vi "Saveissue.vi"() -> ()   [LabVIEW 2011]
panel:
  out "Acquiring Data":bool
  in  "Cancel Acquisition":bool caption="Cancel\nAcquisition"
  in  "Horizontal bin":i32=1
  in  "Vertical bin":i32=1
  in  "Number in series":i32=3
  out "Calculated Exposure Value":sgl format="%.4f"
  out "Return from CheckTimings":u32
  in  "Stop":bool
  in  "Time between captures (s)":dbl
  in  "Number of captures":i32=1
  in  "Run Kinetic":bool caption="Run\nKinetic"
  in  "Start Delay (s)":u32
  out "Image Array":i32[](array[numeric]) caption="Array"
  out "Intensity Graph":i32[][](graph)
  out "SetTriggerMode":u32
  out "SetVSSpeed":u32
  out "SetHSSpeed":u32
  out "SetExposureTime":u32
  in  "Exposure Time (secs)":sgl=0.1 format="%.2f"
  out "SetImage":u32
  out "SetReadMode":u32
  out "SetAcquisition Mode":u32
  out "X Pixels":i32
  out "Y Pixels":i32
  out "GetDetector":u32
  out "Total number of pixels":i32
  out "error out":errorcluster
  in  "Base Path":path=path "D:/Andor/data"
  in  "File Name":string="test"
  in  "File #":i32=1
  out "Sample Output File":string="D:\\Andor\\data\\test_1.sif"
  out "Current":i32 caption="Current Capture Number"
  out "Next Image Time":timestamp
  in  "error in (no error)":errorcluster
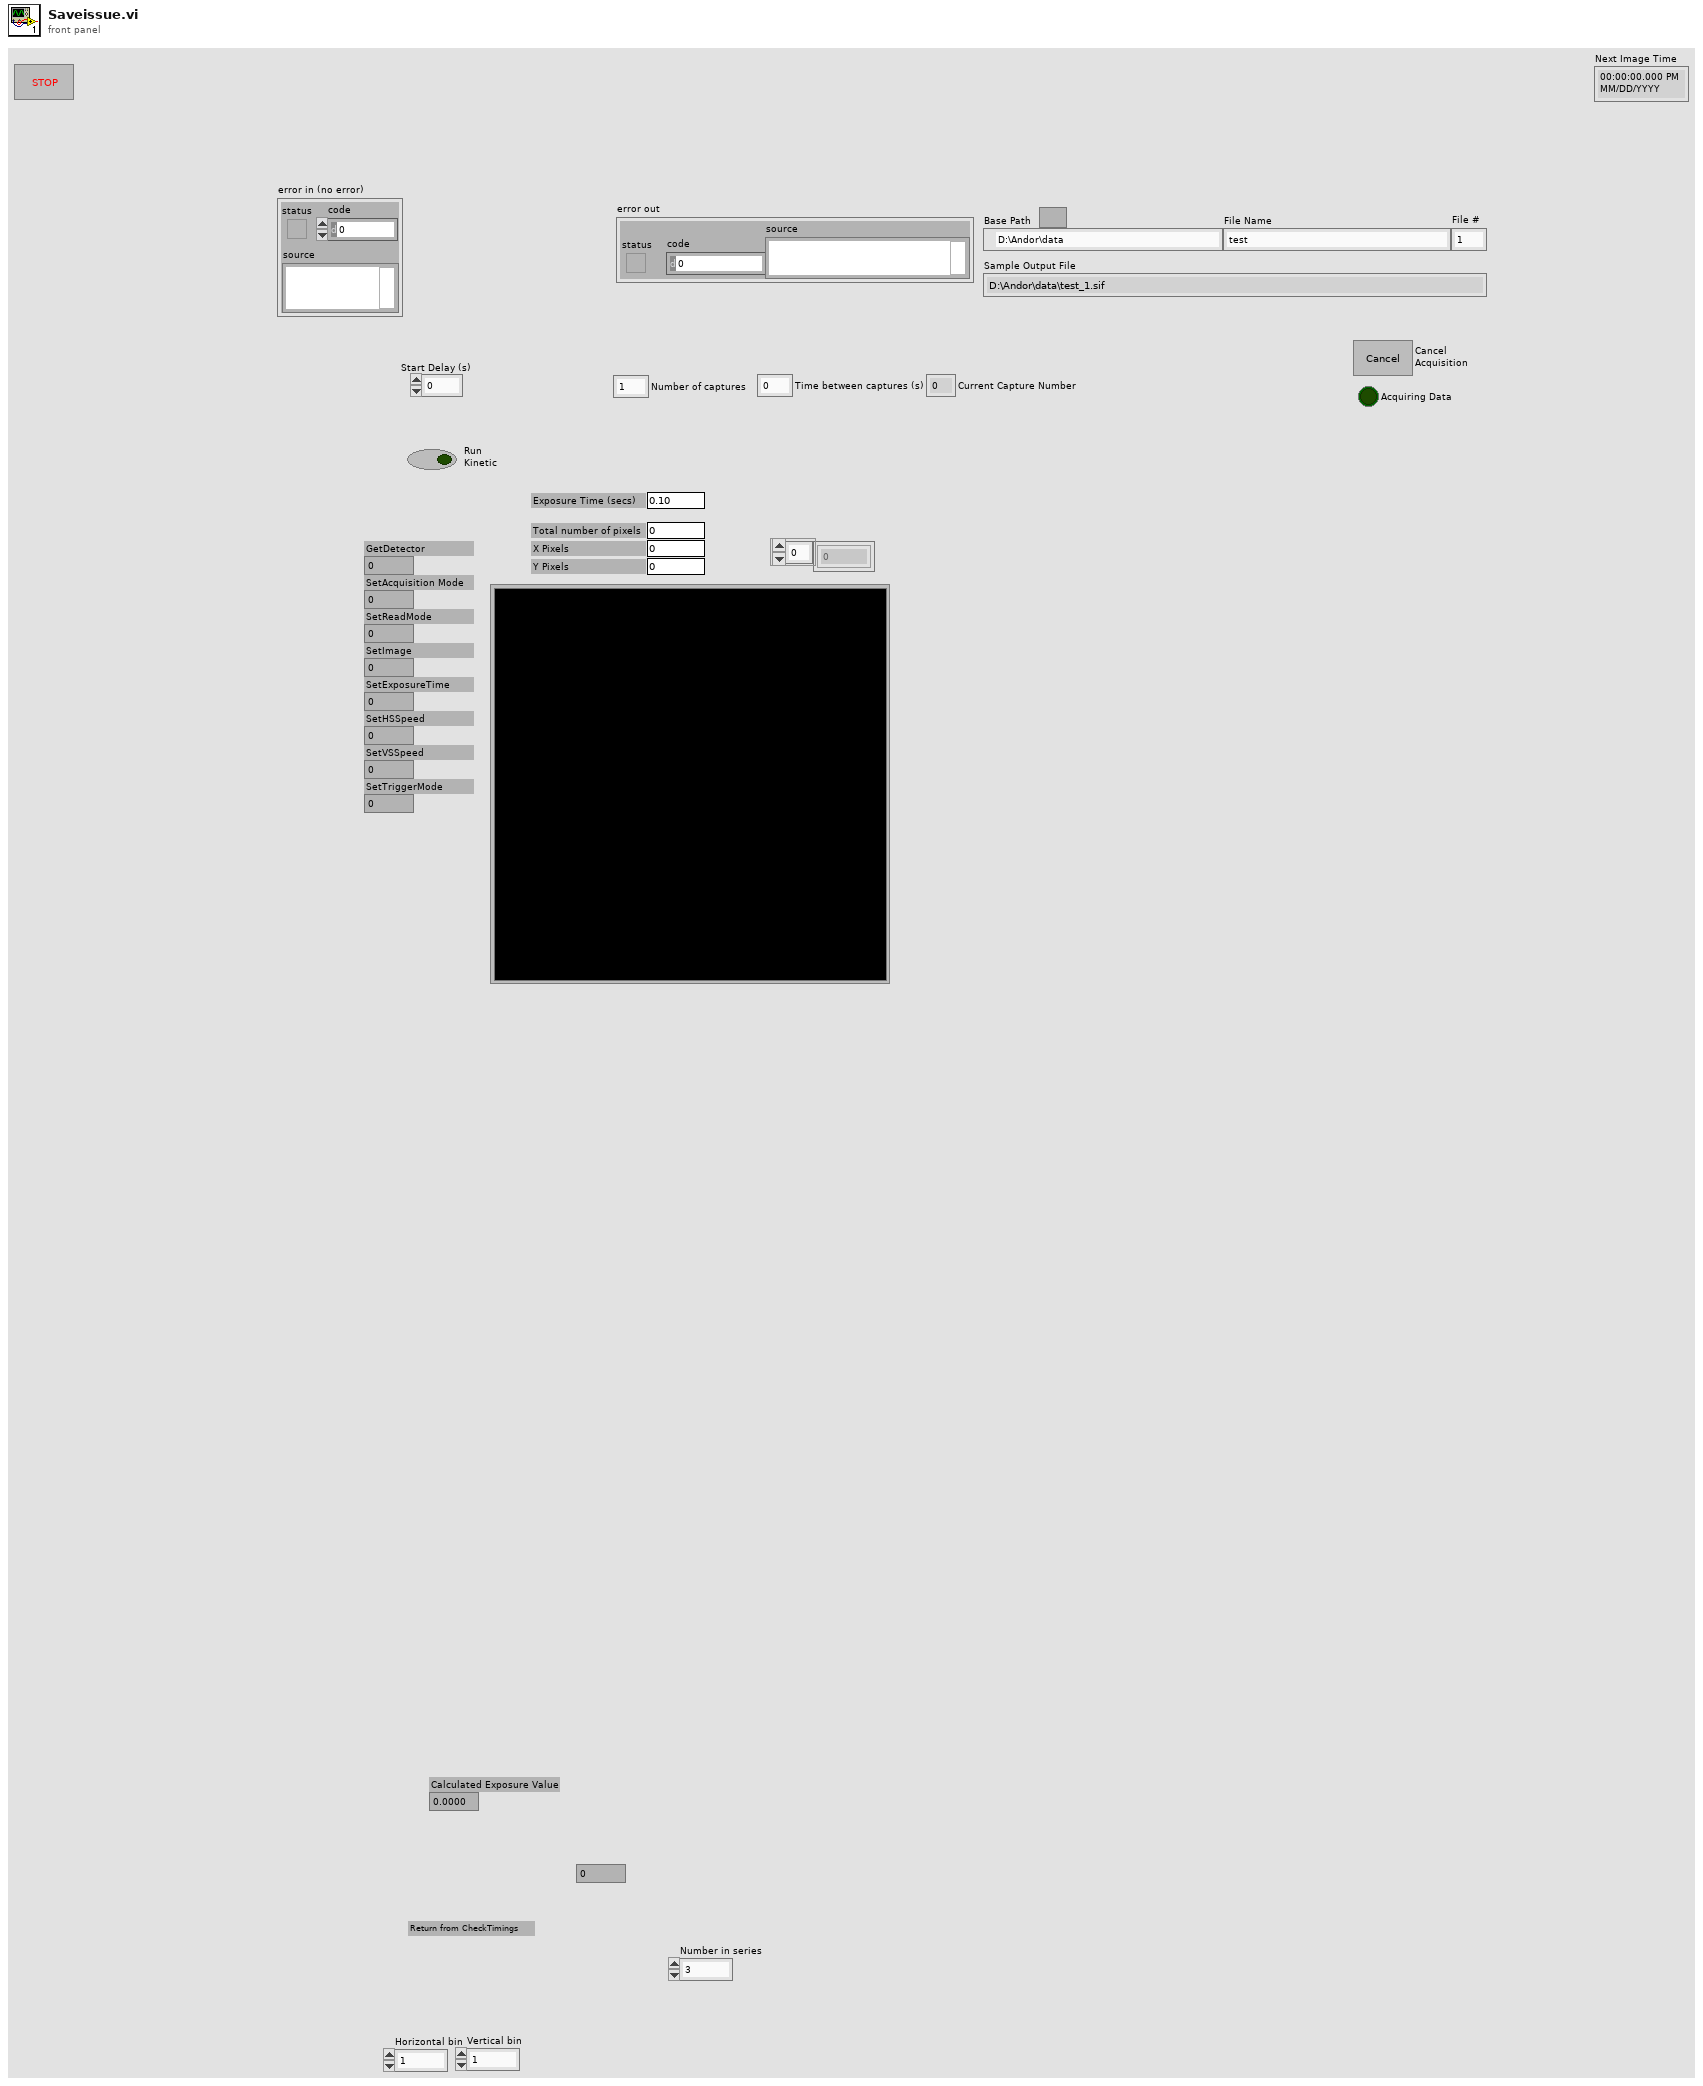
[diagram p1: front panel]
types:
  T1 = typedef "Error Code Enum typedef.ctl" = enum32{"N/A (0)", "DRV_ERROR_CODES", "DRV_SUCCESS", "DRV_VXDNOTINSTALLED", "DRV_ERROR_SCAN", "DRV_ERROR_CHECK_SUM", "DRV_ERROR_FILELOAD", "DRV_UNKNOWN_FUNC", "DRV_ERROR_VXD_INIT", "DRV_ERROR_ADDRESS", "DRV_ERROR_PAGELOCK", "DRV_ERROR_PAGEUNLOCK", "DRV_ERROR_BOARDTEST", "DRV_ERROR_ACK", "DRV_ERROR_UP_FIFO", "DRV_ERROR_PATTERN", "N/A (16)", "DRV_ACQUISITION_ERRORS", "DRV_ACQ_BUFFER", "DRV_ACQ_DOWNFIFO_FULL", "DRV_PROC_UNKONWN_INSTRUCTION", "DRV_ILLEGAL_OP_CODE", "DRV_KINETIC_TIME_NOT_MET", "DRV_ACCUM_TIME_NOT_MET", "DRV_NO_NEW_DATA", "N/A (25)", "DRV_SPOOLERROR", "N/A (27)", "N/A (28)", "N/A (29)", "N/A (30)", "N/A (31)", "N/A (32)", "DRV_TEMPERATURE_CODES", "DRV_TEMPERATURE_OFF", "DRV_TEMPERATURE_NOT_STABILIZED", "DRV_TEMPERATURE_STABILIZED", "DRV_TEMPERATURE_NOT_REACHED", "DRV_TEMPERATURE_OUT_RANGE", "DRV_TEMPERATURE_NOT_SUPPORTED", "DRV_TEMPERATURE_DRIFT", "N/A (41)", "N/A (42)", "N/A (43)", "N/A (44)", "N/A (45)", "N/A (46)", "N/A (47)", "N/A (48)", "DRV_GENERAL_ERRORS", "DRV_INVALID_AUX", "DRV_COF_NOTLOADED", "DRV_FPGAPROG", "DRV_FLEXERROR", "DRV_GPIBERROR", "N/A (55)", "N/A (56)", "N/A (57)", "N/A (58)", "N/A (59)", "N/A (60)", "N/A (61)", "N/A (62)", "N/A (63)", "DRV_DATATYPE", "DRV_DRIVER_ERRORS", "DRV_P1INVALID", "DRV_P2INVALID", "DRV_P3INVALID", "DRV_P4INVALID", "DRV_INIERROR", "DRV_COFERROR", "DRV_ACQUIRING", "DRV_IDLE", "DRV_TEMPCYCLE", "DRV_NOT_INITIALIZED", "DRV_P5INVALID", "DRV_P6INVALID", "DRV_INVALID_MODE", "DRV_INVALID_FILTER", "DRV_I2CERRORS", "DRV_I2CDEVNOTFOUND", "DRV_I2CTIMEOUT", "DRV_P7INVALID", "N/A (84)", "N/A (85)", "N/A (86)", "N/A (87)", "N/A (88)", "N/A (89)", "DRV_IOCERROR", "DRV_VRMVERSIONERROR"}
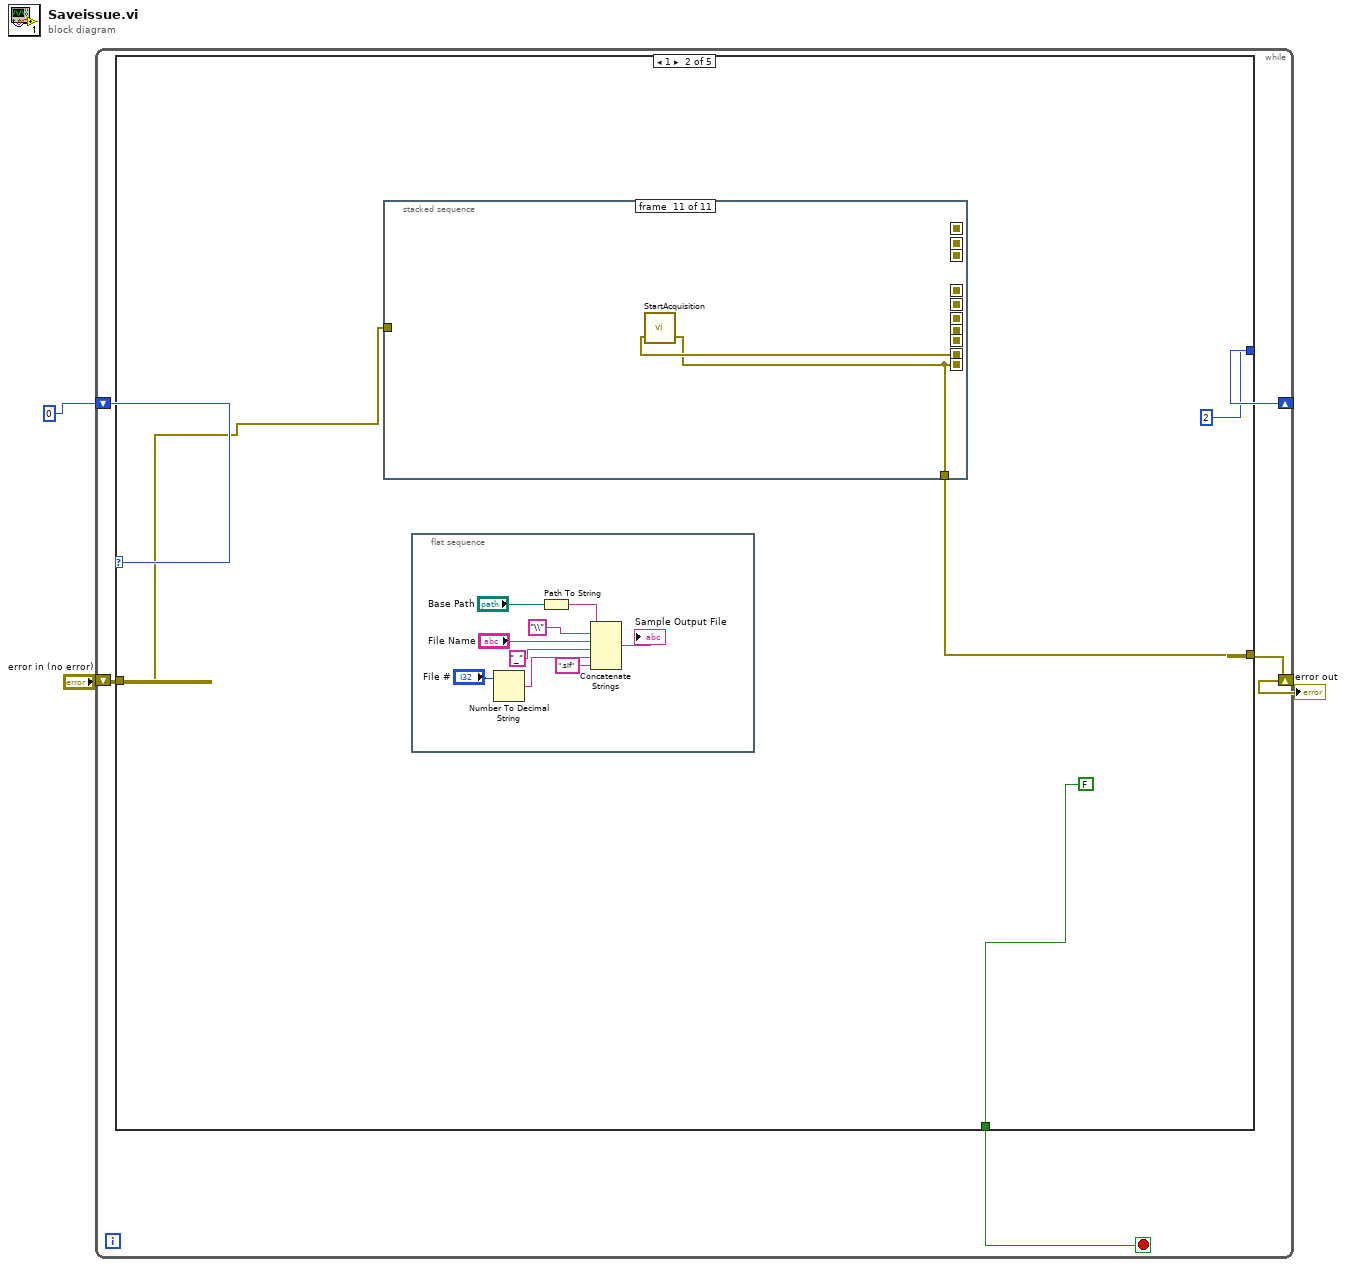
[diagram p0: block diagram]
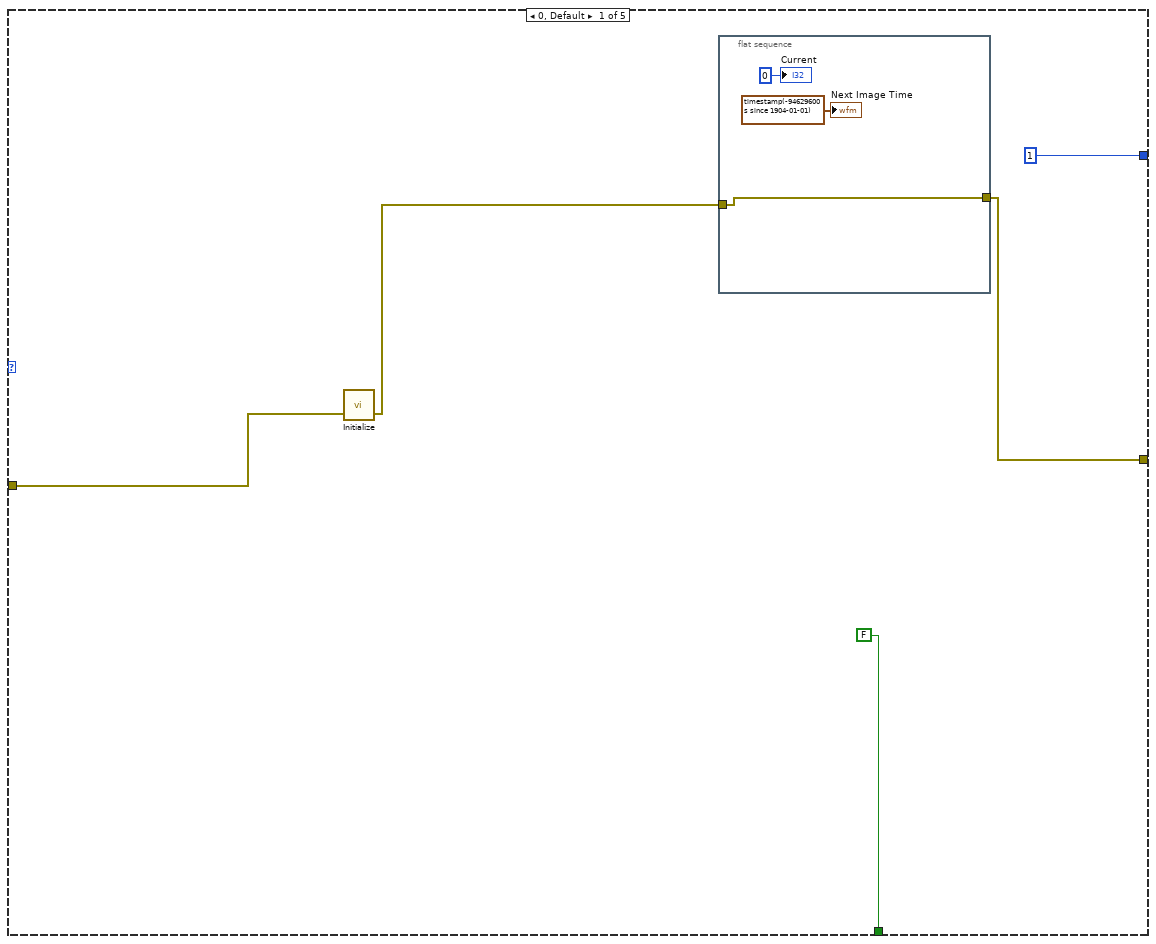
[diagram p2: hidden frame]
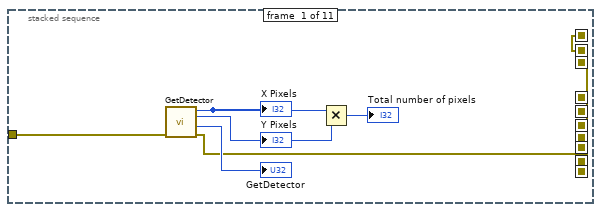
[diagram p3: hidden frame]
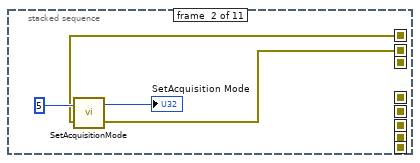
[diagram p4: hidden frame]
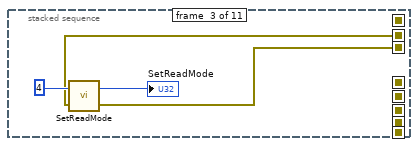
[diagram p5: hidden frame]
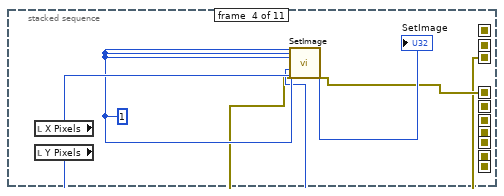
[diagram p6: hidden frame]
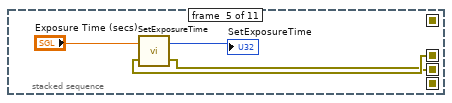
[diagram p7: hidden frame]
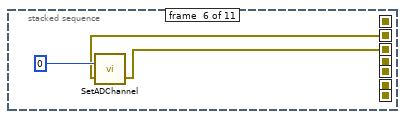
[diagram p8: hidden frame]
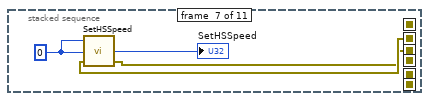
[diagram p9: hidden frame]
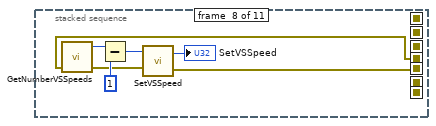
[diagram p10: hidden frame]
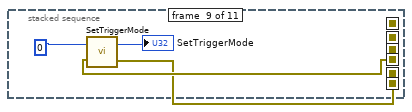
[diagram p11: hidden frame]
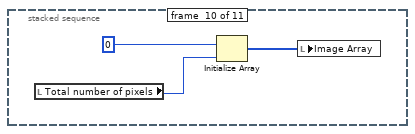
[diagram p12: hidden frame]
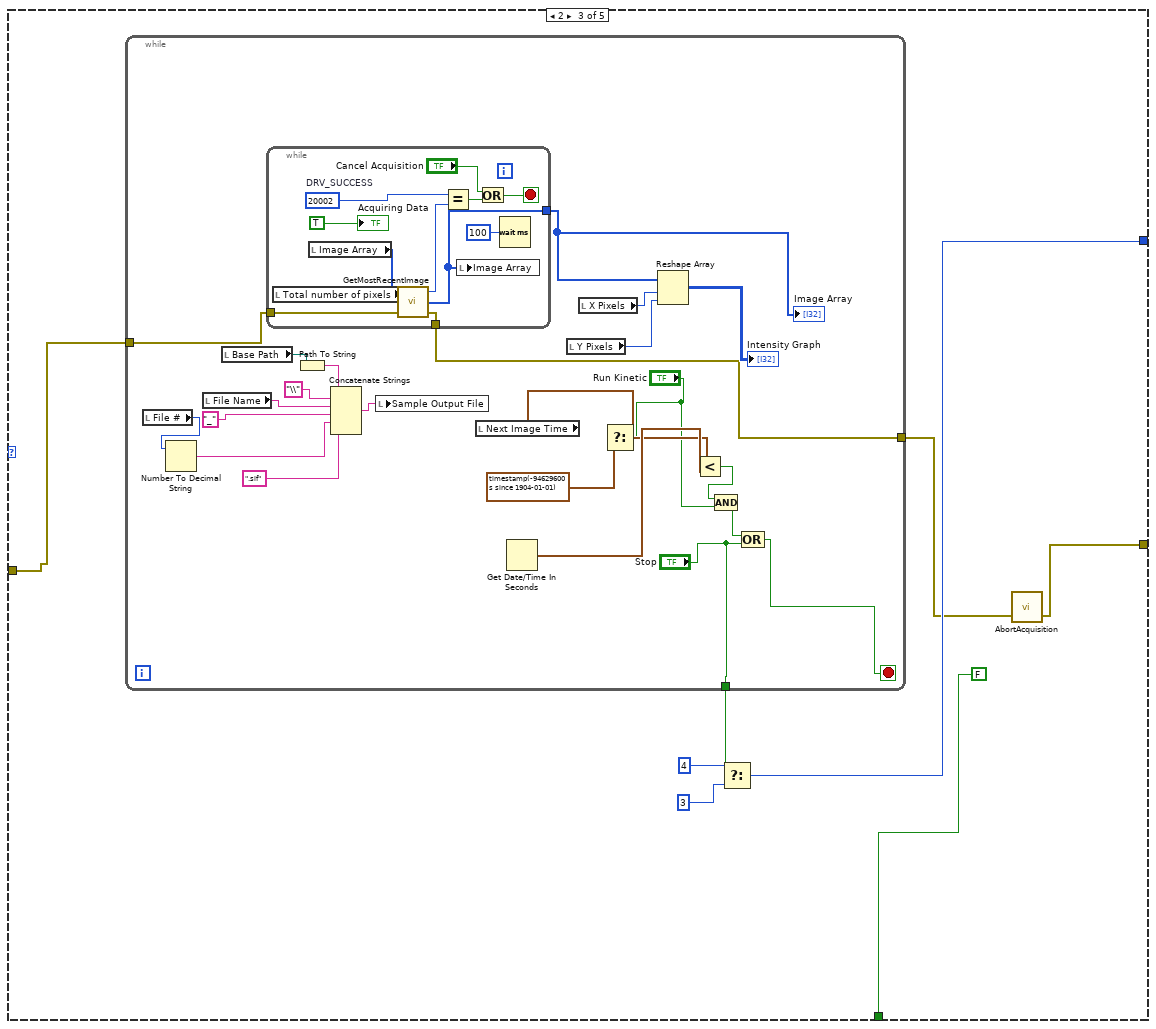
[diagram p13: hidden frame]
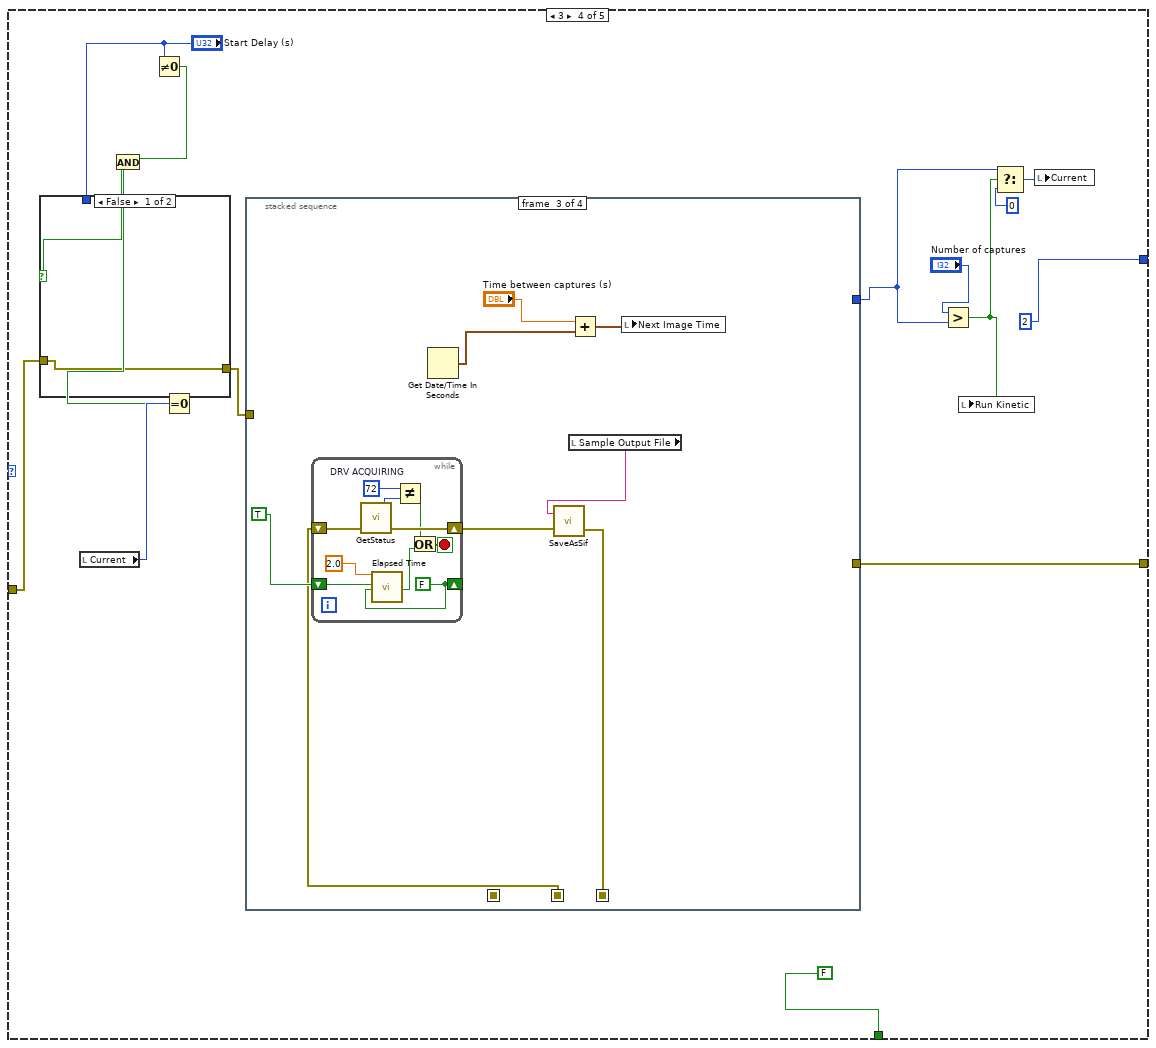
[diagram p14: hidden frame]
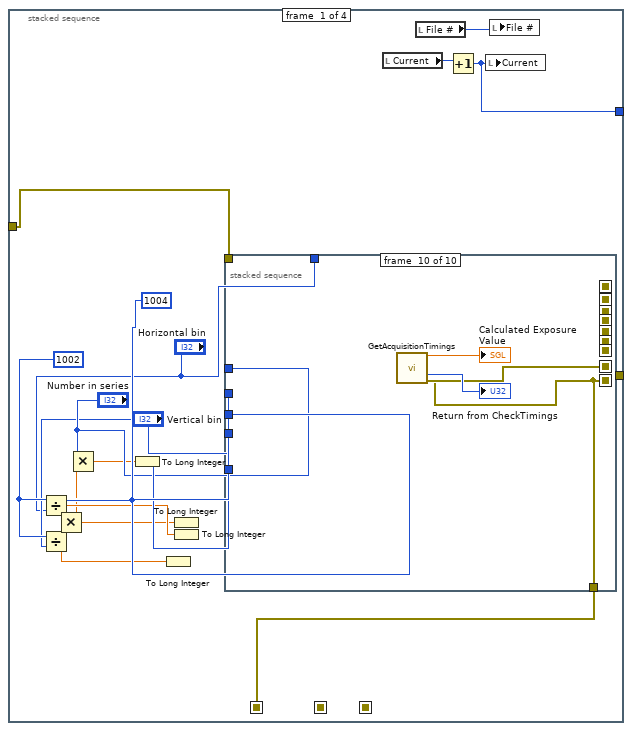
[diagram p15: hidden frame]
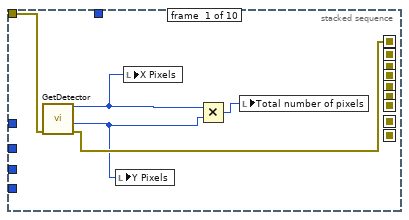
[diagram p16: hidden frame]
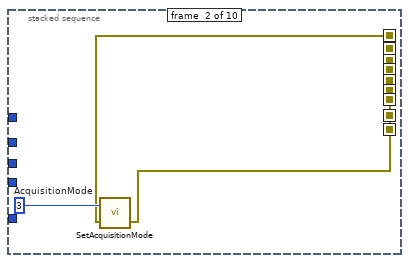
[diagram p17: hidden frame]
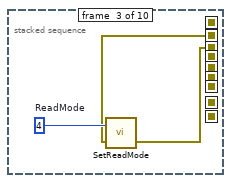
[diagram p18: hidden frame]
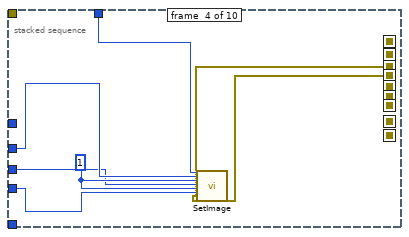
[diagram p19: hidden frame]
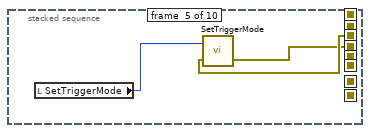
[diagram p20: hidden frame]
diagram:
  n1 = while {
    shift-right: [w5] -> _
    shift-left: 0 -> [w8]
    shift-right: [w6] -> w1
    shift-left: "error in (no error)" -> [w7]
    stop <- w4 stop-if-true
    n2 = case shown="1" w8 {
      tunnel: w7 -> [w10 w19 w78 w122 w269]
      tunnel: [w12 w17 w80 w123 w268] -> w6
      tunnel: [1 2 w81 2 4] -> w5
      tunnel: [FALSE FALSE FALSE FALSE TRUE] -> w4
      frame 0, Default {
        n3 = call <userlib>:"Initialize.vi"("error in (no error)"=w10) -> ("error out"=w9:errorcluster)  [unwired: 1 in, 1 out]
        n4 = flat-sequence {
          tunnel: w9 -> [w14]
          tunnel: [w14] -> w12
          frame #0 {
            "Current" <- 0 ("Current")
            "Next Image Time" <- timestamp(-94629600 s since 1904-01-01) ("Last Image Time")
          }
        }
      }
      frame 1 {
        n5 = stacked-sequence {
          seq-local: [w30 _ _ _ _ _ _ _ _ _ _] -> [_ w37 _ _ _ _ _ _ _ _ _]
          seq-local: [_ w36 _ _ _ _ _ _ _ _ _] -> [_ _ w41 _ _ _ _ _ _ _ _]
          seq-local: [_ _ w40 _ _ _ _ _ _ _ _] -> [_ _ _ w44 _ _ _ _ _ _ _]
          seq-local: [_ _ _ w45 _ _ _ _ _ _ _] -> [_ _ _ _ w51 _ _ _ _ _ _]
          seq-local: [_ _ _ _ w50 _ _ _ _ _ _] -> [_ _ _ _ _ w55 _ _ _ _ _]
          seq-local: [_ _ _ _ _ w54 _ _ _ _ _] -> [_ _ _ _ _ _ w58 _ _ _ _]
          seq-local: [_ _ _ _ _ _ w57 _ _ _ _] -> [_ _ _ _ _ _ _ w63 _ _ _]
          seq-local: [_ _ _ _ _ _ _ w61 _ _ _] -> [_ _ _ _ _ _ _ _ w69 _ _]
          seq-local: [_ _ _ _ _ _ _ _ w68 _ _] -> [_ _ _ _ _ _ _ _ _ _ w76]
          seq-local: [_ _ _ _ _ _ _ _ _ _ w75] -> [_ _ _ _ _ _ _ _ _ _ _]
          tunnel: w19 -> [w31 _ _ _ _ _ _ _ _ _ _]
          tunnel: [_ _ _ _ _ _ _ _ _ _ w75] -> w17
          frame #0 {
            n6 = call <userlib>:"GetDetector.vi"("error in (no error)"=w31) -> ("error out"=w30:errorcluster, "DLL error code"=→"GetDetector":u32, "ypixels"=w34:i32, "xpixels"=w33:i32)  [unwired: 3 out]
            "X Pixels" <- w33
            "Y Pixels" <- w34
            n7 = Multiply(x=w33, y=w34) -> (x*y=→"Total number of pixels":i32)
          }
          frame #1 {
            n8 = call <userlib>:"SetAcquisitionMode.vi"("error in (no error)"=w37, "mode"=u16 5 ("AcquisitionMode")) -> ("error out"=w36:errorcluster, "DLL error code"=→"SetAcquisition Mode":u32)
          }
          frame #2 {
            n9 = call <userlib>:"SetReadMode.vi"("error in (no error)"=w41, "mode"=u16 4 ("ReadMode")) -> ("error out"=w40:errorcluster, "DLL error code"=→"SetReadMode":u32)
          }
          frame #3 {
            w48 = 1
            n10 = local read "X Pixels"() -> (w49:i32)
            n11 = local read "Y Pixels"() -> (w46:i32)
            n12 = call <userlib>:"SetImage.vi"("hbin"=w48, "vbin"=w48, "hstart"=w48, "hend"=w49, "vstart"=w48, "vend"=w46, "error in (no error)"=w44) -> ("DLL error code"=→"SetImage":u32, "error out"=w45:errorcluster)  [unwired: 19 out]
          }
          frame #4 {
            n13 = call <userlib>:"SetExposureTime.vi"("error in (no error)"=w51, "time"="Exposure Time (secs)") -> ("error out"=w50:errorcluster, "DLL error code"=→"SetExposureTime":u32)
          }
          frame #5 {
            n14 = call <userlib>:"SetADChannel.vi"("error in (no error)"=w55, "channel"=0) -> ("error out"=w54:errorcluster)  [unwired: 1 out]
          }
          frame #6 {
            w59 = 0 ("input param")
            n15 = call <userlib>:"SetHSSpeed.vi"("error in (no error)"=w58, "index"=w59, "type"=w59) -> ("error out"=w57:errorcluster, "DLL error code"=→"SetHSSpeed":u32)  [unwired: 1 out]
          }
          frame #7 {
            n16 = call <userlib>:"GetNumberVSSpeeds.vi"("error in (no error)"=w63) -> ("error out"=w62:errorcluster, "number"=w66:i32)  [unwired: 3 out]
            n17 = Subtract(x=w66, y=1) -> (x-y=w64:i32)
            n18 = call <userlib>:"SetVSSpeed.vi"("error in (no error)"=w62, "index"=w64) -> ("error out"=w61:errorcluster, "DLL error code"=→"SetVSSpeed":u32)
          }
          frame #8 {
            n19 = call <userlib>:"SetTriggerMode.vi"("error in (no error)"=w69, "mode"=0) -> ("error out"=w68:errorcluster, "DLL error code"=→"SetTriggerMode":u32)
          }
          frame #9 {
            n20 = local read "Total number of pixels"() -> (w73:i32)
            n21 = Initialize Array(0, w73) -> (w72:i32[])
            n22 = local write "Image Array"(w72) -> ()
          }
          frame #10 {
            n23 = call <userlib>:"StartAcquisition.vi"("error in (no error)"=w76) -> ("error out"=w75:errorcluster)  [unwired: 1 in, 1 out]
          }
        }
        n24 = flat-sequence {
          frame #0 {
            n25 = Number To Decimal String(number="File #") -> (decimal integer string=w28:string)  [unwired: 1 in]
            n26 = Path To String(path="Base Path") -> (string=w25:string)
            n27 = Concatenate Strings(w25, "\\" ("string"), "File Name", "_" ("string"), w28, ".sif" ("string")) -> (→"Sample Output File":string)
          }
        }
      }
      frame 2 {
        n28 = while {
          tunnel: ["Stop"] -> w79
          tunnel: w78 -> [w86]
          tunnel: [w85] -> w77
          stop <- w88 stop-if-true
          n29 = local read "File #"() -> (w99:i32)
          n30 = Number To Decimal String(number=w99) -> (decimal integer string=w98:string)  [unwired: 1 in]
          n31 = local read "File Name"() -> (w101:string)
          n32 = local read "Base Path"() -> (w104:path)
          n33 = while {
            tunnel: [w111] -> w108
            tunnel: w86 -> [w116]
            tunnel: [w109] -> w85
            stop <- w113 stop-if-true
            w110 = 20002  # DRV_SUCCESS
            n34 = local read "Total number of pixels"() -> (w120:i32)
            n35 = local read "Image Array"() -> (w119:i32[])
            n36 = call <userlib>:"GetMostRecentImage.vi"("error in (no error)"=w116, "size"=w120, "array"=w119) -> ("error out"=w109:errorcluster, "array"=w111:i32[], "DLL error code"=w117:u32)
            n37 = Equal?(x=w110, y=w117) -> (x = y?=w114:bool)
            n38 = local write "Image Array"(w111) -> ()
            n39 = Or(x="Cancel Acquisition", y=w114) -> (x .or. y?=w113:bool)
            n40 = Wait (ms)(milliseconds to wait=u32 100) -> ()  [unwired: 1 out]
            "Acquiring Data" <- TRUE
          }
          "Image Array" <- w108
          n41 = Path To String(path=w104) -> (string=w103:string)
          n42 = Concatenate Strings(w103, "\\" ("string"), w101, "_" ("string"), w98, ".sif" ("string")) -> (w96:string)
          n43 = local write "Sample Output File"(w96) -> ()
          n44 = local read "Next Image Time"() -> (w92:timestamp)
          n45 = Get Date/Time In Seconds() -> (seconds since 1Jan1904=w95:timestamp)
          n46 = local read "Y Pixels"() -> (w106:i32)
          n47 = local read "X Pixels"() -> (w107:i32)
          n48 = Select(t=w92, s="Run Kinetic", f=timestamp(-94629600 s since 1904-01-01) ("Last Image Time")) -> (s? t:f=w94:timestamp)
          n49 = Reshape Array(w108, w107, w106) -> (→"Intensity Graph":i32[][])
          n50 = Less?(x=w94, y=w95) -> (x < y?=w91:bool)
          n51 = Compound Arithmetic op=AND(w91, "Run Kinetic") -> (w89:bool)
          n52 = Compound Arithmetic op=OR(w89, "Stop") -> (w88:bool)
        }
        n53 = Select(t=4, s=w79, f=3 ("t")) -> (s? t:f=w81:i32)
        n54 = call <userlib>:"AbortAcquisition.vi"("error in (no error)"=w77) -> ("error out"=w80:errorcluster)  [unwired: 1 in, 1 out]
      }
      frame 3 {
        n55 = local read "Current"() -> (w132:i32)
        n56 = Not Equal To 0?(x="Start Delay (s)") -> (x != 0?=w134:bool)
        n57 = Equal To 0?(x=w132) -> (x = 0?=w131:bool)
        n58 = And(x=w134, y=w131) -> (x .and. y?=w133:bool)
        n59 = case shown="False" w133 {
          tunnel: "Start Delay (s)" -> [_ w261]
          tunnel: w122 -> [w259 w260]
          tunnel: [w259 w260] -> w121
          frame False {
          }
          frame True {
            n60 = flat-sequence {
              tunnel: w261 -> [w262]
              tunnel: w260 -> [_]
              frame #0 {
                n61 = for {
                  N: w262 -> [w264]
                  i -> [w263]
                  n62 = Subtract(x=w264, y=w263) -> ()  [unwired: 1 out]
                  n63 = Wait (ms)(milliseconds to wait=u32 1000) -> ()  [unwired: 1 out]
                }
              }
            }
          }
        }
        n64 = stacked-sequence {
          seq-local: [w136 _ _ _] -> [_ w189 _ _]
          seq-local: [_ w188 _ _] -> [_ _ w191 _]
          seq-local: [_ _ w193 _] -> [_ _ _ w209]
          tunnel: [w148 _ _ _] -> w129
          tunnel: w121 -> [w137 _ _ _]
          tunnel: [_ _ _ w208] -> w123
          frame #0 {
            w146 = 1002
            w147 = 1004
            n65 = Divide(x=w147, y="Horizontal bin") -> (x/y=w141:dbl)
            n66 = Divide(x=w146, y="Vertical bin") -> (x/y=w140:dbl)
            n67 = Multiply(x=w141, y=w140) -> (x*y=w139:dbl)
            n68 = Multiply(x="Number in series", y=w139) -> (x*y=w138:dbl)
            n69 = To Long Integer(number=w138) -> (32bit integer=w145:i32)
            n70 = To Long Integer(number=w140) -> ()  [unwired: 1 out]
            n71 = To Long Integer(number=w139) -> ()  [unwired: 1 out]
            n72 = To Long Integer(number=w141) -> ()  [unwired: 1 out]
            n73 = stacked-sequence {
              seq-local: [w154 _ _ _ _ _ _ _ _ _] -> [_ w157 _ _ _ _ _ _ _ _]
              seq-local: [_ w156 _ _ _ _ _ _ _ _] -> [_ _ w160 _ _ _ _ _ _ _]
              seq-local: [_ _ w159 _ _ _ _ _ _ _] -> [_ _ _ w163 _ _ _ _ _ _]
              seq-local: [_ _ _ w162 _ _ _ _ _ _] -> [_ _ _ _ w171 _ _ _ _ _]
              seq-local: [_ _ _ _ w170 _ _ _ _ _] -> [_ _ _ _ _ w174 _ _ _ _]
              seq-local: [_ _ _ _ _ w173 _ _ _ _] -> [_ _ _ _ _ _ _ w177 _ _]
              seq-local: [_ _ _ _ _ _ _ w175 _ _] -> [_ _ _ _ _ _ _ _ w182 _]
              seq-local: [_ _ _ _ _ _ _ _ w181 _] -> [_ _ _ _ _ _ _ _ _ w185]
              seq-local: [_ _ _ _ _ _ _ _ _ w184] -> [_ _ _ _ _ _ _ _ _ _]
              tunnel: "Horizontal bin" -> [_ _ _ w167 _ _ _ _ _ _]
              tunnel: "Vertical bin" -> [_ _ _ w166 _ _ _ _ _ _]
              tunnel: w147 -> [_ _ _ w165 _ _ _ _ _ _]
              tunnel: "Number in series" -> [_ _ _ _ _ _ _ _ w183 _]
              tunnel: w146 -> [_ _ _ w164 _ _ _ _ _ _]
              tunnel: w145 -> [_ _ _ _ _ _ _ _ _ _]
              tunnel: w137 -> [w155 _ _ _ _ _ _ _ _ _]
              tunnel: [_ _ _ _ _ _ _ _ _ w184] -> w136
              frame #0 {
                n74 = call <userlib>:"GetDetector.vi"("error in (no error)"=w155) -> ("error out"=w154:errorcluster, "DLL error code"=w152:u32, "xpixels"=w153:i32)  [unwired: 4 out]
                n75 = local write "Y Pixels"(w152) -> ()
                n76 = local write "X Pixels"(w153) -> ()
                n77 = Multiply(x=w153, y=w152) -> (x*y=w151:u32)
                n78 = local write "Total number of pixels"(w151) -> ()
              }
              frame #1 {
                w158 = u16 3  # AcquisitionMode
                n79 = call <userlib>:"SetAcquisitionMode.vi"("error in (no error)"=w157, "mode"=w158) -> ("error out"=w156:errorcluster)  [unwired: 1 out]
              }
              frame #2 {
                w161 = u16 4  # ReadMode
                n80 = call <userlib>:"SetReadMode.vi"("error in (no error)"=w160, "mode"=w161) -> ("error out"=w159:errorcluster)  [unwired: 1 out]
              }
              frame #3 {
                w168 = 1
                n81 = call <userlib>:"SetImage.vi"("hbin"=w167, "vbin"=w166, "hstart"=w168, "hend"=w165, "vstart"=w168, "vend"=w164, "error in (no error)"=w163) -> ("error out"=w162:errorcluster)  [unwired: 20 out]
              }
              frame #4 {
                n82 = local read "SetTriggerMode"() -> (w169:u32)
                n83 = call <userlib>:"SetTriggerMode.vi"("error in (no error)"=w171, "mode"=w169) -> ("error out"=w170:errorcluster)  [unwired: 1 out]
              }
              frame #5 {
                n84 = local read "Exposure Time (secs)"() -> (w172:sgl)
                n85 = call <userlib>:"SetExposureTime.vi"("error in (no error)"=w174, "time"=w172) -> ("error out"=w173:errorcluster)  [unwired: 1 out]
              }
              frame #6 {
              }
              frame #7 {
                n86 = call <userlib>:"GetNumberVSSpeeds.vi"("error in (no error)"=w177) -> ("error out"=w176:errorcluster, "number"=w178:i32)  [unwired: 3 out]
                n87 = Subtract(x=w178, y=1) -> (x-y=w180:i32)
                n88 = call <userlib>:"SetVSSpeed.vi"("error in (no error)"=w176, "index"=w180) -> ("error out"=w175:errorcluster)  [unwired: 1 out]
              }
              frame #8 {
                n89 = call <userlib>:"SetNumberKinetics.vi"("error in (no error)"=w182, "number"=w183) -> ("error out"=w181:errorcluster)  [unwired: 1 out]
              }
              frame #9 {
                n90 = call <userlib>:"GetAcquisitionTimings.vi"("error in (no error)"=w185) -> ("exposure"=→"Calculated Exposure Value":sgl, "DLL error code"=→"Return from CheckTimings":u32, "error out"=w184:errorcluster)  [unwired: 3 in, 9 out]
              }
            }
            n91 = local read "Current"() -> (w149:i32)
            n92 = local read "File #"() -> (w150:i32)
            n93 = Increment(x=w149) -> (x+1=w148:i32)
            n94 = local write "Current"(w148) -> ()
            n95 = local write "File #"(w150) -> ()
          }
          frame #1 {
            n96 = call <userlib>:"StartAcquisition.vi"("error in (no error)"=w189) -> ("error out"=w188:errorcluster)  [unwired: 1 in, 1 out]
          }
          frame #2 {
            n97 = while {
              shift-right: [w204] -> w190
              shift-left: w191 -> [w205]
              shift-right: [w198] -> _
              shift-left: TRUE ("Reset") -> [w199]
              stop <- w203 stop-if-true
              w198 = FALSE
              w207 = u16 72  # DRV ACQUIRING
              n98 = call <userlib>:"GetStatus.vi"("error in (no error)"=w205) -> ("error out"=w204:errorcluster, "status"=w206:T1)  [unwired: 3 out]
              n99 = call "Elapsed Time"("Time Target (s)"=2.0, "Reset"=w199, "Auto Reset"=w198) -> ("Time has Elapsed"=w201:bool)  [unwired: 2 in, 14 out]
              n100 = Not Equal?(x=w207, y=w206) -> (x != y?=w202:bool)
              n101 = Or(x=w202, y=w201) -> (x .or. y?=w203:bool)
            }
            n102 = Get Date/Time In Seconds() -> (seconds since 1Jan1904=w196:timestamp)
            n103 = local read "Sample Output File"() -> (w194:string)
            n104 = call <userlib>:"SaveAsSif.vi"("error in (no error)"=w190, "path"=w194) -> ("error out"=w193:errorcluster)  [unwired: 1 out]
            n105 = Add(x="Time between captures (s)", y=w196) -> (x+y=w195:timestamp)
            n106 = local write "Next Image Time"(w195) -> ()
          }
          frame #3 {
            w216 = 1004
            w215 = 1002
            n107 = local read "Number in series"() -> (w217:i32)
            n108 = local read "Horizontal bin"() -> (w218:i32)
            n109 = Divide(x=w216, y=w218) -> (x/y=w213:dbl)
            n110 = To Long Integer(number=w213) -> ()  [unwired: 1 out]
            n111 = local read "Vertical bin"() -> (w219:i32)
            n112 = Divide(x=w215, y=w219) -> (x/y=w212:dbl)
            n113 = Multiply(x=w213, y=w212) -> (x*y=w211:dbl)
            n114 = Multiply(x=w217, y=w211) -> (x*y=w210:dbl)
            n115 = To Long Integer(number=w210) -> (32bit integer=w214:i32)
            n116 = To Long Integer(number=w212) -> ()  [unwired: 1 out]
            n117 = To Long Integer(number=w211) -> ()  [unwired: 1 out]
            n118 = stacked-sequence {
              seq-local: [w223 _ _ _ _ _ _ _ _ _ _] -> [_ w226 _ _ _ _ _ _ _ _ _]
              seq-local: [_ w225 _ _ _ _ _ _ _ _ _] -> [_ _ w229 _ _ _ _ _ _ _ _]
              seq-local: [_ _ w228 _ _ _ _ _ _ _ _] -> [_ _ _ w232 _ _ _ _ _ _ _]
              seq-local: [_ _ _ w231 _ _ _ _ _ _ _] -> [_ _ _ _ w240 _ _ _ _ _ _]
              seq-local: [_ _ _ _ w239 _ _ _ _ _ _] -> [_ _ _ _ _ w243 _ _ _ _ _]
              seq-local: [_ _ _ _ _ w242 _ _ _ _ _] -> [_ _ _ _ _ _ _ w246 _ _ _]
              seq-local: [_ _ _ _ _ _ _ w244 _ _ _] -> [_ _ _ _ _ _ _ _ w251 _ _]
              seq-local: [_ _ _ _ _ _ _ _ w250 _ _] -> [_ _ _ _ _ _ _ _ _ w256 _]
              seq-local: [_ _ _ _ _ _ _ _ _ w255 _] -> [_ _ _ _ _ _ _ _ _ _ w258]
              seq-local: [_ _ _ _ _ _ _ _ _ _ w257] -> [_ _ _ _ _ _ _ _ _ _ _]
              tunnel: w218 -> [_ _ _ w236 _ _ _ _ _ _ _]
              tunnel: w219 -> [_ _ _ w235 _ _ _ _ _ _ _]
              tunnel: w216 -> [_ _ _ w234 _ _ _ _ _ _ _]
              tunnel: w217 -> [_ _ _ _ _ _ _ _ w252 _ _]
              tunnel: w215 -> [_ _ _ w233 _ _ _ _ _ _ _]
              tunnel: w214 -> [_ _ _ _ _ _ _ _ _ _ _]
              tunnel: w209 -> [w224 _ _ _ _ _ _ _ _ _ _]
              tunnel: [_ _ _ _ _ _ _ _ _ _ w257] -> _
              tunnel: [_ _ _ _ _ _ _ _ _ _ w257] -> w208
              frame #0 {
                n119 = call <userlib>:"GetDetector.vi"("error in (no error)"=w224) -> ("error out"=w223:errorcluster, "ypixels"=w221:i32, "xpixels"=w222:i32)  [unwired: 4 out]
                n120 = local write "X Pixels"(w222) -> ()
                n121 = local write "Y Pixels"(w221) -> ()
                n122 = Multiply(x=w222, y=w221) -> (x*y=w220:i32)
                n123 = local write "Total number of pixels"(w220) -> ()
              }
              frame #1 {
                w227 = u16 3  # AcquisitionMode
                n124 = call <userlib>:"SetAcquisitionMode.vi"("error in (no error)"=w226, "mode"=w227) -> ("error out"=w225:errorcluster)  [unwired: 1 out]
              }
              frame #2 {
                w230 = u16 4  # ReadMode
                n125 = call <userlib>:"SetReadMode.vi"("error in (no error)"=w229, "mode"=w230) -> ("error out"=w228:errorcluster)  [unwired: 1 out]
              }
              frame #3 {
                w237 = 1
                n126 = call <userlib>:"SetImage.vi"("hbin"=w236, "vbin"=w235, "hstart"=w237, "hend"=w234, "vstart"=w237, "vend"=w233, "error in (no error)"=w232) -> ("error out"=w231:errorcluster)  [unwired: 20 out]
              }
              frame #4 {
                n127 = local read "SetTriggerMode"() -> (w238:u32)
                n128 = call <userlib>:"SetTriggerMode.vi"("error in (no error)"=w240, "mode"=w238) -> ("error out"=w239:errorcluster)  [unwired: 1 out]
              }
              frame #5 {
                n129 = local read "Exposure Time (secs)"() -> (w241:sgl)
                n130 = call <userlib>:"SetExposureTime.vi"("error in (no error)"=w243, "time"=w241) -> ("error out"=w242:errorcluster)  [unwired: 1 out]
              }
              frame #6 {
              }
              frame #7 {
                n131 = call <userlib>:"GetNumberVSSpeeds.vi"("error in (no error)"=w246) -> ("error out"=w245:errorcluster, "number"=w247:i32)  [unwired: 3 out]
                n132 = Subtract(x=w247, y=1) -> (x-y=w249:i32)
                n133 = call <userlib>:"SetVSSpeed.vi"("error in (no error)"=w245, "index"=w249) -> ("error out"=w244:errorcluster)  [unwired: 1 out]
              }
              frame #8 {
                n134 = call <userlib>:"SetNumberKinetics.vi"("error in (no error)"=w251, "number"=w252) -> ("error out"=w250:errorcluster)  [unwired: 1 out]
              }
              frame #9 {
                n135 = call <userlib>:"GetAcquisitionTimings.vi"("error in (no error)"=w256) -> ("exposure"=w254:sgl, "DLL error code"=w253:u32, "error out"=w255:errorcluster)  [unwired: 3 in, 9 out]
                n136 = local write "Return from CheckTimings"(w253) -> ()
                n137 = local write "Calculated Exposure Value"(w254) -> ()
              }
              frame #10 {
                n138 = call <userlib>:"StartAcquisition.vi"("error in (no error)"=w258) -> ("error out"=w257:errorcluster)  [unwired: 2 out]
              }
            }
          }
        }
        n139 = Greater?(x="Number of captures", y=w129) -> (0:w127:bool)
        n140 = local write "Run Kinetic"(w127) -> ()
        n141 = Select(t=w129, s=w127, f=0) -> (s? t:f=w126:i32)
        n142 = local write "Current"(w126) -> ()
      }
      frame 4 {
        n143 = call <userlib>:"ShutDown.vi"("error in (no error)"=w269) -> ("error out"=w268:errorcluster)  [unwired: 1 in, 1 out]
      }
    }
  }
  "error out" <- w1
